vi "KnowPose.vi"() -> ()   [LabVIEW 2019]
uses:
  refnums.vi
  dsinstructions.vi
  sensors.vi
  dsdata.vi
  autoinfo.vi
panel:
  out "Y Position (in)":dbl
  out "X Position (in)":dbl
  out "Robot Position":cluster{dbl[], dbl[]}(graph)
  out "Heading (deg)":dbl format="%#_13g"
  in  "Plot Data":bool
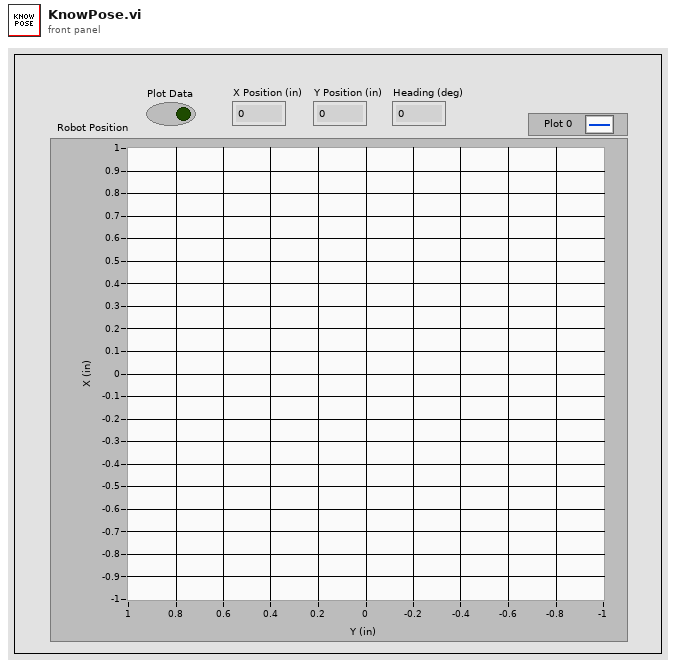
[diagram p1: front panel]
types:
  T1 = typedef "WPI_MotorControlDeviceRef.ctl" = cluster{"DeviceStatus":errorcluster, "Type":T2, "PWM":cluster{"PWM Channel":T3, "DeadBand":T4}, "CAN":cluster{"Device Number":u8, "SetOutput VI Ref":variant, "GetOutput VI Ref":variant, "Enable VI Ref":variant, "Disable VI Ref":variant, "Data":variant}, "Invert":bool, "DIO PWM":cluster{"PWM \"Enable\" Channel":T3, "DIOChannel":T5, "PWM Rate":dbl}}
  T2 = typedef "WPI_MotorControlType.ctl" = enum16{"PWM", "CAN", "DIO PWM"}
  T3 = typedef "FPGA_DIOPWMChannel.ctl" = enum8{"PWM 0", "PWM 1", "PWM 2", "PWM 3", "PWM 4", "PWM 5", "PWM 6", "PWM 7", "PWM 8", "PWM 9", "PWM MXP 0", "PWM MXP 1", "PWM MXP 2", "PWM MXP 3", "PWM MXP 4", "PWM MXP 5", "PWM MXP 6", "PWM MXP 7", "PWM MXP 8", "PWM MXP 9", "Invalid"}
  T4 = typedef "WPI_PWMDeadband.ctl" = cluster{"Name":string, "maxPositivePwm":i32, "minPositivePwm":i32, "centerPwm":i32, "maxNegativePwm":i32, "minNegativePwm":i32, "angularRange":u16}
  T5 = typedef "FPGA_DIOChannel.ctl" = enum8{"DIO 0", "DIO 1", "DIO 2", "DIO 3", "DIO 4", "DIO 5", "DIO 6", "DIO 7", "DIO 8", "DIO 9", "DIO MXP 0", "DIO MXP 1", "DIO MXP 2", "DIO MXP 3", "DIO MXP 4", "DIO MXP 5", "DIO MXP 6", "DIO MXP 7", "DIO MXP 8", "DIO MXP 9", "DIO MXP 10", "DIO MXP 11", "DIO MXP 12", "DIO MXP 13", "DIO MXP 14", "DIO MXP 15", "SPI Port CS1", "SPI Port CS2", "SPI Port CS3", "SPI Port MISO", "SPI Port MOSI", "Invalid"}
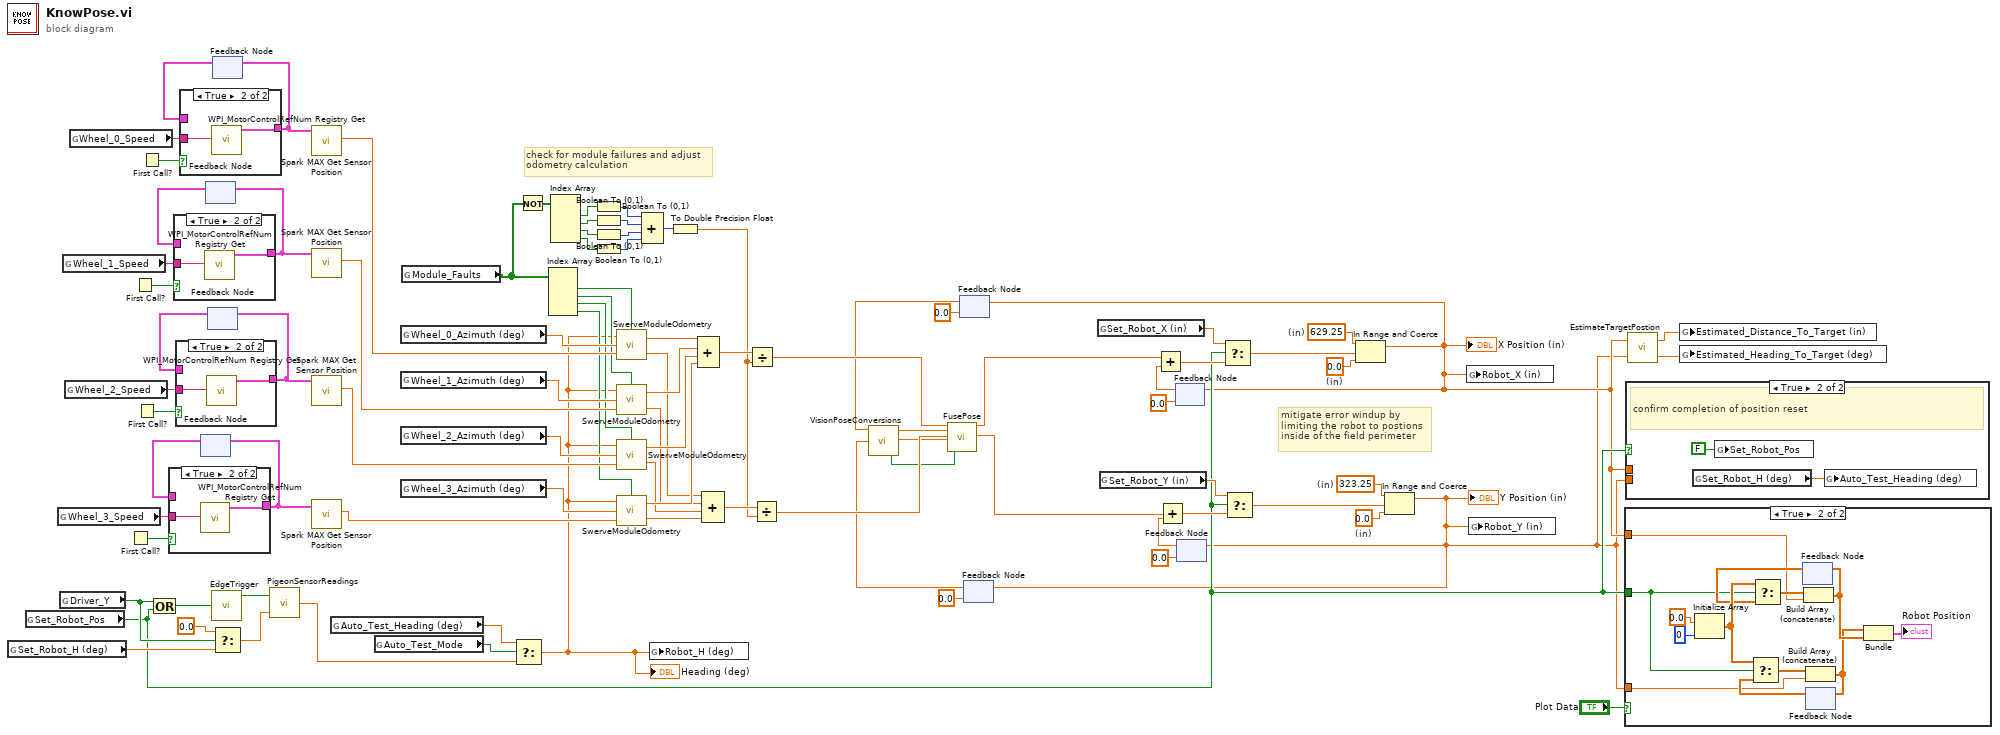
[diagram p0: block diagram]
diagram:
  w4 = 323.25  # (in)
  w5 = 0.0  # (in)
  w6 = 629.25  # (in)
  w7 = 0.0  # (in)
  # "mitigate error windup by\nlimiting the robot to postions\ninside of the field perimeter"
  # "check for module failures and adjust\nodometry calculation"
  n1 = global read "sensors.vi" "Set_Robot_H (deg)"() -> (w48:dbl)
  n2 = global read "sensors.vi" "Set_Robot_Pos"() -> (w23:bool)
  n3 = global read "refnums.vi" "Wheel_3_Speed"() -> (w80:string)
  n4 = global read "dsinstructions.vi" "Driver_Y"() -> (w47:bool)
  n5 = global read "refnums.vi" "Wheel_1_Speed"() -> (w86:string)
  n6 = global read "refnums.vi" "Wheel_2_Speed"() -> (w83:string)
  n7 = global read "refnums.vi" "Wheel_0_Speed"() -> (w89:string)
  n8 = First Call?() -> (First Call?: T/F=w82:bool)
  n9 = First Call?() -> (First Call?: T/F=w88:bool)
  n10 = First Call?() -> (First Call?: T/F=w85:bool)
  n11 = First Call?() -> (First Call?: T/F=w91:bool)
  n12 = Compound Arithmetic op=OR(w47, w23) -> (w46:bool)
  n13 = feedback #1() -> (w81:T1)  [unwired: 1 in]
  n14 = case shown="True" w82 {
    tunnel: [w92 w93] -> w77
    tunnel: w81 -> [w92 _]
    tunnel: w80 -> [_ w94]
    frame False {
    }
    frame True {
      n15 = call <vilib>:"WPI_MotorControlRefNum Registry Get.vi"("refnum name"=w94) -> ("MotorControlDevRef"=w93:T1)  [unwired: 9 in, 1 out]
    }
  }
  n16 = feedback-in #1(w77) -> ()
  n17 = feedback #2() -> (w87:T1)  [unwired: 1 in]
  n18 = case shown="True" w88 {
    tunnel: [w95 w96] -> w79
    tunnel: w87 -> [w95 _]
    tunnel: w86 -> [_ w97]
    frame False {
    }
    frame True {
      n19 = call <vilib>:"WPI_MotorControlRefNum Registry Get.vi"("refnum name"=w97) -> ("MotorControlDevRef"=w96:T1)  [unwired: 9 in, 1 out]
    }
  }
  n20 = feedback-in #2(w79) -> ()
  n21 = feedback #3() -> (w84:T1)  [unwired: 1 in]
  n22 = case shown="True" w85 {
    tunnel: [w98 w99] -> w78
    tunnel: w84 -> [w98 _]
    tunnel: w83 -> [_ w100]
    frame False {
    }
    frame True {
      n23 = call <vilib>:"WPI_MotorControlRefNum Registry Get.vi"("refnum name"=w100) -> ("MotorControlDevRef"=w99:T1)  [unwired: 9 in, 1 out]
    }
  }
  n24 = feedback-in #3(w78) -> ()
  n25 = call "EdgeTrigger.vi"("Input Signal"=w46) -> ("Rising Edge Trigger"=w45:bool)  [unwired: 2 out]
  n26 = feedback #4() -> (w90:T1)  [unwired: 1 in]
  n27 = case shown="True" w91 {
    tunnel: [w101 w102] -> w76
    tunnel: w90 -> [w101 _]
    tunnel: w89 -> [_ w103]
    frame False {
    }
    frame True {
      n28 = call <vilib>:"WPI_MotorControlRefNum Registry Get.vi"("refnum name"=w103) -> ("MotorControlDevRef"=w102:T1)  [unwired: 9 in, 1 out]
    }
  }
  n29 = feedback-in #4(w76) -> ()
  n30 = Select(t=0.0 ("f"), s=w47, f=w48) -> (s? t:f=w50:dbl)
  n31 = call "PigeonSensorReadings.vi"("Reset Yaw (deg)"=w50, "Reset Yaw"=w45) -> ("Yaw (deg)"=w26:dbl)
  n32 = call <vilib>:"Spark MAX Get Sensor Position.vi"("MotorControlDevRef in"=w76) -> ("Sensor Position"=w74:dbl)  [unwired: 7 in, 3 out]
  n33 = call <vilib>:"Spark MAX Get Sensor Position.vi"("MotorControlDevRef in"=w79) -> ("Sensor Position"=w72:dbl)  [unwired: 7 in, 3 out]
  n34 = call <vilib>:"Spark MAX Get Sensor Position.vi"("MotorControlDevRef in"=w78) -> ("Sensor Position"=w71:dbl)  [unwired: 7 in, 3 out]
  n35 = call <vilib>:"Spark MAX Get Sensor Position.vi"("MotorControlDevRef in"=w77) -> ("Sensor Position"=w43:dbl)  [unwired: 7 in, 3 out]
  n36 = global read "autoinfo.vi" "Auto_Test_Heading (deg)"() -> (w24:dbl)
  n37 = global read "dsdata.vi" "Auto_Test_Mode"() -> (w25:bool)
  n38 = global read "sensors.vi" "Wheel_0_Azimuth (deg)"() -> (w73:dbl)
  n39 = global read "sensors.vi" "Wheel_1_Azimuth (deg)"() -> (w70:dbl)
  n40 = global read "sensors.vi" "Wheel_2_Azimuth (deg)"() -> (w69:dbl)
  n41 = global read "sensors.vi" "Wheel_3_Azimuth (deg)"() -> (w44:dbl)
  n42 = global read "sensors.vi" "Module_Faults"() -> (w42:bool[])
  n43 = Select(t=w24, s=w25, f=w26) -> (s? t:f=w1:dbl)
  "Heading (deg)" <- w1
  n44 = Not(x=w42) -> (.not. x?=w41:bool[])
  n45 = Index Array(array=w42) -> (element #1=w30:bool, element #2=w29:bool, element #3=w28:bool, element #4=w27:bool)  [unwired: 4 in]
  n46 = Index Array(array=w41) -> (element #1=w40:bool, element #2=w39:bool, element #3=w38:bool, element #4=w37:bool)  [unwired: 4 in]
  n47 = Boolean To (0,1)(Boolean=w40) -> (0, 1=w36:i16)
  n48 = Boolean To (0,1)(Boolean=w39) -> (0, 1=w35:i16)
  n49 = Boolean To (0,1)(Boolean=w38) -> (0, 1=w34:i16)
  n50 = Boolean To (0,1)(Boolean=w37) -> (0, 1=w33:i16)
  n51 = call "SwerveModuleOdometry.vi"("Module Fault"=w30, "Wheel Distance (native)"=w74, "Wheel Azimuth (deg)"=w73, "Robot Heading(deg)"=w1) -> ("Delta Y (in)"=w59:dbl, "Delta X (in)"=w68:dbl)
  n52 = call "SwerveModuleOdometry.vi"("Module Fault"=w29, "Wheel Distance (native)"=w72, "Wheel Azimuth (deg)"=w70, "Robot Heading(deg)"=w1) -> ("Delta Y (in)"=w60:dbl, "Delta X (in)"=w67:dbl)
  n53 = call "SwerveModuleOdometry.vi"("Module Fault"=w28, "Wheel Distance (native)"=w71, "Wheel Azimuth (deg)"=w69, "Robot Heading(deg)"=w1) -> ("Delta Y (in)"=w61:dbl, "Delta X (in)"=w66:dbl)
  n54 = call "SwerveModuleOdometry.vi"("Module Fault"=w27, "Wheel Distance (native)"=w43, "Wheel Azimuth (deg)"=w44, "Robot Heading(deg)"=w1) -> ("Delta Y (in)"=w62:dbl, "Delta X (in)"=w65:dbl)
  n55 = Compound Arithmetic op=ADD(w36, w35, w34, w33) -> (w32:i16)
  n56 = global write "sensors.vi" "Robot_H (deg)"(w1) -> ()
  n57 = To Double Precision Float(number=w32) -> (double precision float=w31:dbl)
  n58 = Compound Arithmetic op=ADD(w68, w67, w66, w65) -> (w64:dbl)
  n59 = Compound Arithmetic op=ADD(w59, w60, w61, w62) -> (w63:dbl)
  n60 = Divide(x=w64, y=w31) -> (x/y=w22:dbl)
  n61 = Divide(x=w63, y=w31) -> (x/y=w19:dbl)
  n62 = feedback #5(0.0 ("Set_Robot_X (in)")) -> (w14:dbl)
  n63 = feedback #6(0.0 ("Set_Robot_Y (in)")) -> (w15:dbl)
  n64 = call "VisionPoseConversions.vi"("Current X Estimate (in)"=w14, "Current Y Estimate (in)"=w15) -> ("deltaX (in)"=w17:dbl, "deltaY (in)"=w18:dbl, "Synced LimeLight Pose Valid"=w12:bool)  [unwired: 1 in, 1 out]
  n65 = call "FusePose.vi"("Odometry deltaX"=w22, "LimeLight deltaX"=w17, "Odometry deltaY"=w19, "LimeLight deltaY"=w18, "LimeLight Pose Valid"=w12) -> ("Fused deltaX"=w21:dbl, "Fused deltaY"=w20:dbl)  [unwired: 13 in]
  n66 = global read "sensors.vi" "Set_Robot_X (in)"() -> (w55:dbl)
  n67 = global read "sensors.vi" "Set_Robot_Y (in)"() -> (w51:dbl)
  n68 = feedback #7(0.0) -> (w58:dbl)
  n69 = Add(x=w21, y=w58) -> (x+y=w56:dbl)
  n70 = feedback #8(0.0) -> (w54:dbl)
  n71 = Add(x=w20, y=w54) -> (x+y=w52:dbl)
  n72 = Select(t=w55, s=w23, f=w56) -> (s? t:f=w9:dbl)
  n73 = Select(t=w51, s=w23, f=w52) -> (s? t:f=w3:dbl)
  n74 = In Range and Coerce(upper limit=w6, x=w9, lower limit=w7) -> (coerced(x)=w8:dbl)  [unwired: 1 out]
  "X Position (in)" <- w8
  n75 = feedback-in #5(w8) -> ()
  n76 = feedback-in #7(w8) -> ()
  n77 = In Range and Coerce(upper limit=w4, x=w3, lower limit=w5) -> (coerced(x)=w2:dbl)  [unwired: 1 out]
  "Y Position (in)" <- w2
  n78 = feedback-in #6(w2) -> ()
  n79 = feedback-in #8(w2) -> ()
  n80 = global write "sensors.vi" "Robot_X (in)"(w8) -> ()
  n81 = global write "sensors.vi" "Robot_Y (in)"(w2) -> ()
  n82 = case shown="True" "Plot Data" {
    tunnel: w23 -> [_ w104]
    tunnel: w8 -> [_ w107]
    tunnel: w2 -> [_ w106]
    frame False {
    }
    frame True {
      n83 = Initialize Array(0.0 ("element"), 0 ("dimension size")) -> (w116:dbl[])
      n84 = feedback #9() -> (w112:dbl[])  [unwired: 1 in]
      n85 = Select(t=w116, s=w104, f=w112) -> (s? t:f=w113:dbl[])
      n86 = Build Array (concatenate)(w113, w107) -> (w111:dbl[])
      n87 = feedback-in #9(w111) -> ()
      n88 = feedback #10() -> (w114:dbl[])  [unwired: 1 in]
      n89 = Select(t=w116, s=w104, f=w114) -> (s? t:f=w115:dbl[])
      n90 = Build Array (concatenate)(w115, w106) -> (w110:dbl[])
      n91 = feedback-in #10(w110) -> ()
      n92 = Bundle(w110, w111) -> (→"Robot Position":cluster{dbl[], dbl[]})  [unwired: 1 in]
    }
  }
  n93 = case shown="True" w23 {
    tunnel: w8 -> [_ _]
    tunnel: w2 -> [_ _]
    frame False {
    }
    frame True {
      # "confirm completion of position reset"
      n94 = global read "sensors.vi" "Set_Robot_H (deg)"() -> (w117:dbl)
      n95 = global write "sensors.vi" "Set_Robot_Pos"(FALSE ("Set_Robot_Pos")) -> ()
      n96 = global write "autoinfo.vi" "Auto_Test_Heading (deg)"(w117) -> ()
    }
  }
  n97 = call "EstimateTargetPostion.vi"("Robot Y (in)"=w2, "Robot X (in)"=w8) -> ("Estimated Heading to Target (deg)"=w10:dbl, "Estimated Distance to Target (in)"=w11:dbl)
  n98 = global write "sensors.vi" "Estimated_Distance_To_Target (in)"(w11) -> ()
  n99 = global write "sensors.vi" "Estimated_Heading_To_Target (deg)"(w10) -> ()
